vi "Shoot State.vi"(11 "Trigger":bool) -> (2 "Pullback off":bool, 3 "Release Lock":bool)   [LabVIEW 2013]
uses:
  Control 3.ctl
  <vilib>/Rock Robotics/WPI/Solenoid/Deprecated/WPI_SolenoidSetBool.vi
panel:
  out "Clamp Off":bool
  out "Value":bool
  out "Elapsed Time (s) 2":dbl caption="Elapsed Time (s)"
  out "Pullback On":bool
  out "Lock on":bool
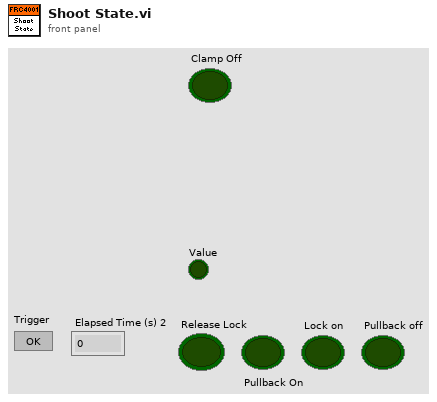
[diagram p1: front panel]
types:
  T1 = typedef "Control 3.ctl" = enum16{"Release Lock", "Pullback On", "Lock On", "Pullback Off"}
  T2 = typedef "WPI_DigitalInputDevRef.ctl" = cluster{"DevStatus":errorcluster, "DIO Channel":T3, "Digital Module":T4}
  T3 = typedef "FPGA_DIOChannel.ctl" = enum8{"DIO 1", "DIO 2", "DIO 3", "DIO 4", "DIO 5", "DIO 6", "DIO 7", "DIO 8", "DIO 9", "DIO 10", "DIO 11", "DIO 12", "DIO 13", "DIO 14", "Invalid"}
  T4 = typedef "FPGA_TypedefDigitalModule.ctl" = enum16{"Digital Module 1", "Digital Module 2"}
  T5 = typedef "WPI_SolenoidDevRef.ctl" = cluster{"DevStatus":errorcluster, "Solenoid Module":T6, "Forward Solenoid Channel":T7, "Reverse Solenoid Channel":T7}
  T6 = typedef "FPGA_TypedefSolenoidModule.ctl" = enum16{"Solenoid Module 1", "Solenoid Module 2"}
  T7 = typedef "WPI_SolenoidChannel.ctl" = enum8{"Solenoid 1", "Solenoid 2", "Solenoid 3", "Solenoid 4", "Solenoid 5", "Solenoid 6", "Solenoid 7", "Solenoid 8", "Invalid"}
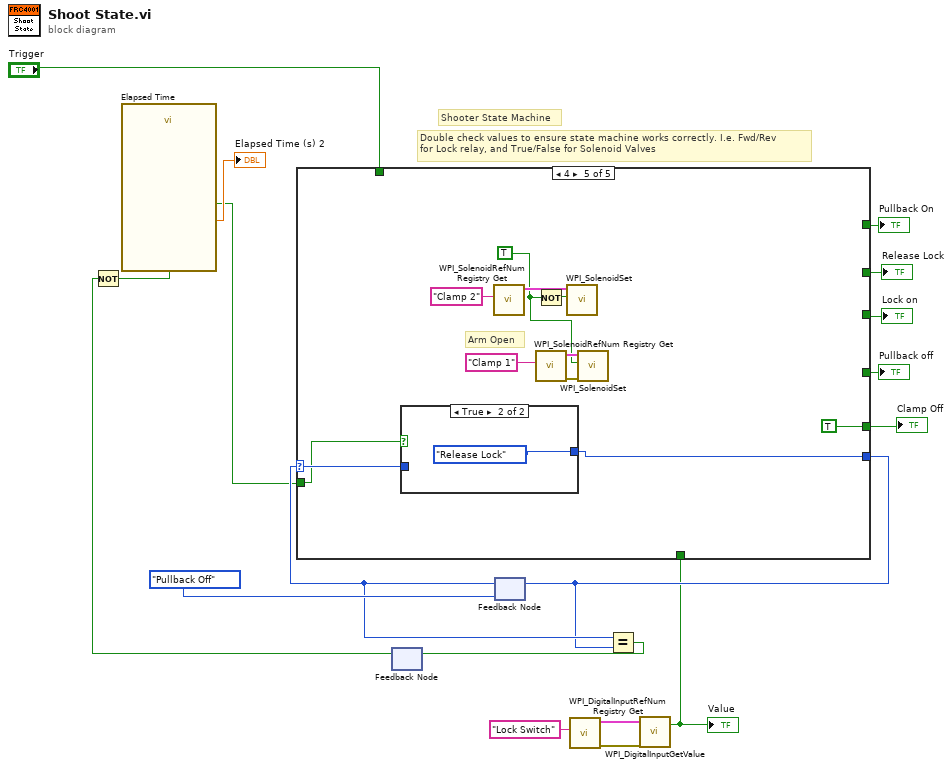
[diagram p0: block diagram]
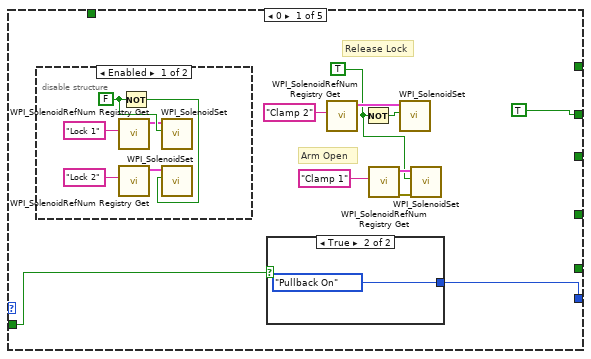
[diagram p2: hidden frame]
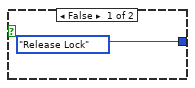
[diagram p4: hidden frame]
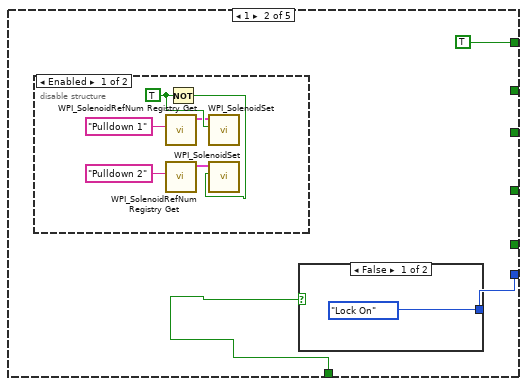
[diagram p5: hidden frame]
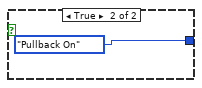
[diagram p7: hidden frame]
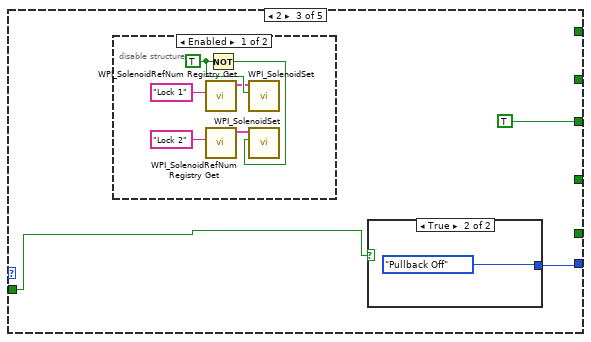
[diagram p8: hidden frame]
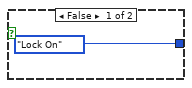
[diagram p10: hidden frame]
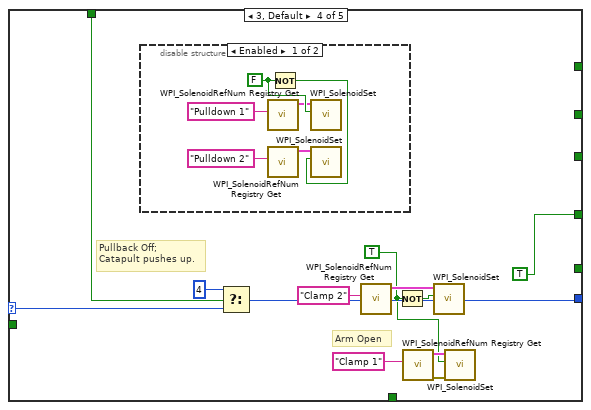
[diagram p11: hidden frame]
diagram:
  # "Double check values to ensure state machine works correctly. I.e. Fwd/Rev\nfor Lock relay, and True/False for Solenoid Valves"
  # "Shooter State Machine"
  n1 = feedback #1() -> (w9:bool)  [unwired: 1 in]
  n2 = Not(x=w9) -> (.not. x?=w7:bool)
  n3 = call "Elapsed Time"("Reset"=w7) -> ("Elapsed Time (s)"=→"Elapsed Time (s) 2":dbl, "Time has Elapsed"=w8:bool)  [unwired: 11 in, 6 out]
  n4 = feedback #2(Control_3."Pullback Off") -> (w13:u32)
  n5 = call <vilib>:"WPI_DigitalInputRefNum Registry Get.vi"("refnum name"="Lock Switch") -> ("error out"=w4:errorcluster, "DigitalInputDevRef"=w5:T2)  [unwired: 9 in]
  n6 = call <vilib>:"WPI_DigitalInputGetValue.vi"("error in (no error)"=w4, "DigitalInputDevRef"=w5) -> ("Value"=w2:bool)  [unwired: 7 in, 2 out]
  "Value" <- w2
  n7 = case shown="4" w13 {
    selector: w13 -> [_ _ _ w69 w79]
    tunnel: [w28 w39 w49 w70 w80] -> w12
    tunnel: [TRUE ("State 0") _ _ _ _] -> w17
    tunnel: [_ TRUE _ _ _] -> w16
    tunnel: [_ _ TRUE _ _] -> w15
    tunnel: [_ _ _ TRUE _] -> w14
    tunnel: w8 -> [w26 _ w48 _ w78]
    tunnel: "Trigger" -> [_ _ _ w67 _]
    tunnel: w2 -> [_ w37 _ _ _]
    tunnel: [_ _ _ _ TRUE] -> w1
    frame 0 {
      w19 = TRUE
      # "Arm Open"
      # "Release Lock"
      n8 = disable-structure shown="Enabled" {
        frame Enabled {
          w34 = FALSE
          n9 = call <vilib>:"WPI_SolenoidRefNum Registry Get.vi"("refnum name"="Lock 1") -> ("SolenoidDevRef"=w30:T5)  [unwired: 9 in, 1 out]
          n10 = call <vilib>:"WPI_SolenoidRefNum Registry Get.vi"("refnum name"="Lock 2") -> ("SolenoidDevRef"=w32:T5)  [unwired: 9 in, 1 out]
          n11 = Not(x=w34) -> (.not. x?=w29:bool)
          n12 = call-poly <vilib>:"WPI_SolenoidSet.vi"("Value"=w34, "SolenoidDevRef"=w30) -> ()  [unwired: 8 in, 2 out]
          n13 = call-poly <vilib>:"WPI_SolenoidSet.vi"("Value"=w29, "SolenoidDevRef"=w32) -> ()  [unwired: 8 in, 2 out]
        }
        frame Disabled {
        }
      }
      n14 = case shown="True" w26 {
        tunnel: [Control_3."Release Lock" Control_3."Pullback On"] -> w28
        frame False {
        }
        frame True {
        }
      }
      n15 = call <vilib>:"WPI_SolenoidRefNum Registry Get.vi"("refnum name"="Clamp 2") -> ("SolenoidDevRef"=w22:T5)  [unwired: 9 in, 1 out]
      n16 = Not(x=w19) -> (.not. x?=w20:bool)
      n17 = call <vilib>:"WPI_SolenoidRefNum Registry Get.vi"("refnum name"="Clamp 1") -> ("error out"=w23:errorcluster, "SolenoidDevRef"=w24:T5)  [unwired: 9 in]
      n18 = call-poly <vilib>:"WPI_SolenoidSet.vi"("Value"=w20, "SolenoidDevRef"=w22) -> ()  [unwired: 8 in, 2 out]
      n19 = call-poly <vilib>:"WPI_SolenoidSet.vi"("error in (no error)"=w23, "Value"=w19, "SolenoidDevRef"=w24) -> ()  [unwired: 7 in, 2 out]
    }
    frame 1 {
      n20 = disable-structure shown="Enabled" {
        frame Enabled {
          w45 = TRUE
          n21 = call <vilib>:"WPI_SolenoidRefNum Registry Get.vi"("refnum name"="Pulldown 1") -> ("SolenoidDevRef"=w41:T5)  [unwired: 9 in, 1 out]
          n22 = call <vilib>:"WPI_SolenoidRefNum Registry Get.vi"("refnum name"="Pulldown 2") -> ("SolenoidDevRef"=w43:T5)  [unwired: 9 in, 1 out]
          n23 = Not(x=w45) -> (.not. x?=w40:bool)
          n24 = call-poly <vilib>:"WPI_SolenoidSet.vi"("Value"=w45, "SolenoidDevRef"=w41) -> ()  [unwired: 8 in, 2 out]
          n25 = call-poly <vilib>:"WPI_SolenoidSet.vi"("Value"=w40, "SolenoidDevRef"=w43) -> ()  [unwired: 8 in, 2 out]
        }
        frame Disabled {
        }
      }
      n26 = case shown="False" w37 {
        tunnel: [Control_3."Lock On" Control_3."Pullback On"] -> w39
        frame False {
        }
        frame True {
        }
      }
    }
    frame 2 {
      n27 = disable-structure shown="Enabled" {
        frame Enabled {
          w56 = TRUE
          n28 = call <vilib>:"WPI_SolenoidRefNum Registry Get.vi"("refnum name"="Lock 1") -> ("SolenoidDevRef"=w52:T5)  [unwired: 9 in, 1 out]
          n29 = call <vilib>:"WPI_SolenoidRefNum Registry Get.vi"("refnum name"="Lock 2") -> ("SolenoidDevRef"=w54:T5)  [unwired: 9 in, 1 out]
          n30 = Not(x=w56) -> (.not. x?=w51:bool)
          n31 = call-poly <vilib>:"WPI_SolenoidSet.vi"("Value"=w56, "SolenoidDevRef"=w52) -> ()  [unwired: 8 in, 2 out]
          n32 = call-poly <vilib>:"WPI_SolenoidSet.vi"("Value"=w51, "SolenoidDevRef"=w54) -> ()  [unwired: 8 in, 2 out]
        }
        frame Disabled {
        }
      }
      n33 = case shown="True" w48 {
        tunnel: [Control_3."Lock On" Control_3."Pullback Off"] -> w49
        frame False {
        }
        frame True {
        }
      }
    }
    frame 3, Default {
      w59 = TRUE
      # "Arm Open"
      # "Pullback Off;\nCatapult pushes up."
      n34 = disable-structure shown="Enabled" {
        frame Enabled {
          w76 = FALSE
          n35 = call <vilib>:"WPI_SolenoidRefNum Registry Get.vi"("refnum name"="Pulldown 1") -> ("SolenoidDevRef"=w72:T5)  [unwired: 9 in, 1 out]
          n36 = call <vilib>:"WPI_SolenoidRefNum Registry Get.vi"("refnum name"="Pulldown 2") -> ("SolenoidDevRef"=w74:T5)  [unwired: 9 in, 1 out]
          n37 = Not(x=w76) -> (.not. x?=w71:bool)
          n38 = call-poly <vilib>:"WPI_SolenoidSet.vi"("Value"=w76, "SolenoidDevRef"=w72) -> ()  [unwired: 8 in, 2 out]
          n39 = call-poly <vilib>:"WPI_SolenoidSet.vi"("Value"=w71, "SolenoidDevRef"=w74) -> ()  [unwired: 8 in, 2 out]
        }
        frame Disabled {
        }
      }
      n40 = Select(t=u32 4, s=w67, f=w69) -> (s? t:f=w70:u32)
      n41 = call <vilib>:"WPI_SolenoidRefNum Registry Get.vi"("refnum name"="Clamp 2") -> ("SolenoidDevRef"=w62:T5)  [unwired: 9 in, 1 out]
      n42 = Not(x=w59) -> (.not. x?=w60:bool)
      n43 = call <vilib>:"WPI_SolenoidRefNum Registry Get.vi"("refnum name"="Clamp 1") -> ("error out"=w63:errorcluster, "SolenoidDevRef"=w64:T5)  [unwired: 9 in]
      n44 = call-poly <vilib>:"WPI_SolenoidSet.vi"("Value"=w60, "SolenoidDevRef"=w62) -> ()  [unwired: 8 in, 2 out]
      n45 = call-poly <vilib>:"WPI_SolenoidSet.vi"("error in (no error)"=w63, "Value"=w59, "SolenoidDevRef"=w64) -> ()  [unwired: 7 in, 2 out]
    }
    frame 4 {
      w81 = TRUE
      # "Arm Open"
      n46 = case shown="True" w78 {
        tunnel: [w88 Control_3."Release Lock"] -> w80
        tunnel: w79 -> [w88 _]
        frame False {
        }
        frame True {
        }
      }
      n47 = call <vilib>:"WPI_SolenoidRefNum Registry Get.vi"("refnum name"="Clamp 2") -> ("SolenoidDevRef"=w84:T5)  [unwired: 9 in, 1 out]
      n48 = Not(x=w81) -> (.not. x?=w82:bool)
      n49 = call <vilib>:"WPI_SolenoidRefNum Registry Get.vi"("refnum name"="Clamp 1") -> ("error out"=w85:errorcluster, "SolenoidDevRef"=w86:T5)  [unwired: 9 in]
      n50 = call-poly <vilib>:"WPI_SolenoidSet.vi"("Value"=w82, "SolenoidDevRef"=w84) -> ()  [unwired: 8 in, 2 out]
      n51 = call-poly <vilib>:"WPI_SolenoidSet.vi"("error in (no error)"=w85, "Value"=w81, "SolenoidDevRef"=w86) -> ()  [unwired: 7 in, 2 out]
    }
  }
  "Release Lock" <- w17
  "Lock on" <- w15
  "Pullback On" <- w16
  "Pullback off" <- w14
  "Clamp Off" <- w1
  n52 = feedback-in #2(w12) -> ()
  n53 = Equal?(x=w13, y=w12) -> (x = y?=w10:bool)
  n54 = feedback-in #1(w10) -> ()
